vi "Create Launcher.vi"(6 "timeout (ms)":i32=5000, 8 "error in":errorcluster, 10 "Loader Info":T1, 11 "gRPC ID in":T3) -> (0 "error out":errorcluster, 3 "gRPC ID out":T3)   [LabVIEW 2021, in "CIFManagerClientWrapper.lvlib"]
uses:
  CIFManagerClientWrapper.lvlib
  <vilib>/gRPC/LabVIEW gRPC Library/Shared/grpcId.ctl
  CIF_Manager_client/RPC Messages/cif_manager_LoaderInfo.ctl
  CIF_Manager_client/RPC Messages/cif_manager_LoaderType.ctl
  CIF_Manager_client/CIF_Manager_client.lvlib
  <vilib>/gRPC/LabVIEW gRPC Library/grpc-lvsupport-release.lvlib
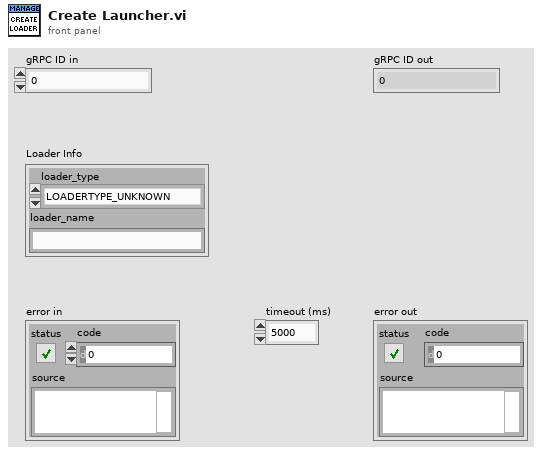
[diagram p1: front panel]
types:
  T1 = typedef "CIF_Manager_client.lvlib/cif_manager_LoaderInfo.ctl" = cluster{"loader_type":T2, "loader_name":string}
  T2 = typedef "CIF_Manager_client.lvlib/cif_manager_LoaderType.ctl" = enum32{"LOADERTYPE_UNKNOWN", "LOADERTYPE_LABVIEW"}
  T3 = typedef "grpc-lvsupport-release.lvlib/grpcId.ctl" = u64
  T4 = typedef "CIF_Manager_client.lvlib/cif_common_Status.ctl" = cluster{"code":i32, "message":string}
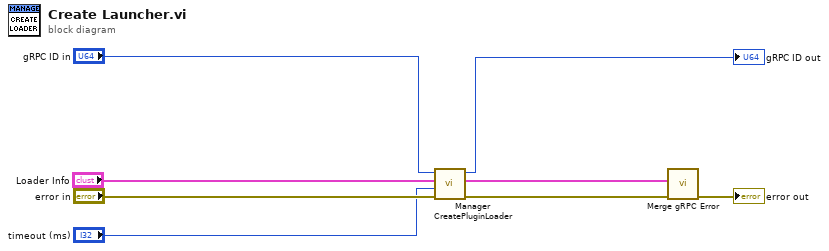
[diagram p0: block diagram]
diagram:
  n1 = call "Manager CreatePluginLoader.vi"("error in"="error in", "timeout (ms)"="timeout (ms)", "Request Data"="Loader Info", "gRPC ID"="gRPC ID in") -> ("error out"=w4:errorcluster, "Response Data"=w2:T4, "gRPC ID out"=→"gRPC ID out":T3)  [unwired: 5 in]
  n2 = call "Merge gRPC Error.vi"("error in (no error)"=w4, "gRPC Error"=w2) -> ("error out"=→"error out":errorcluster)  [unwired: 9 in]
